vi "FeedbackDecode_KalmanElects2Str.vi"(1 "KalmanElects":T1(array[cluster])) -> (0 "KElectStr":string)   [LabVIEW 2020]
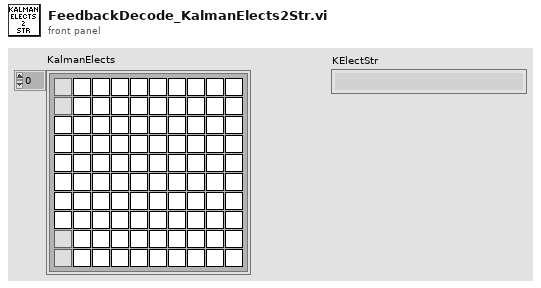
[diagram p1: front panel]
types:
  T1 = cluster{"Boolean 1":bool, "Boolean 2":bool, "Boolean 3":bool, "Boolean 4":bool, "Boolean 5":bool, "Boolean 6":bool, "Boolean 7":bool, "Boolean 8":bool, "Boolean 9":bool, "Boolean 10":bool, "Boolean 11":bool, "Boolean 12":bool, "Boolean 13":bool, "Boolean 14":bool, "Boolean 15":bool, "Boolean 16":bool, "Boolean 17":bool, "Boolean 18":bool, "Boolean 19":bool, "Boolean 20":bool, "Boolean 21":bool, "Boolean 22":bool, "Boolean 23":bool, "Boolean 24":bool, "Boolean 25":bool, "Boolean 26":bool, "Boolean 27":bool, "Boolean 28":bool, "Boolean 29":bool, "Boolean 30":bool, "Boolean 31":bool, "Boolean 32":bool, "Boolean 33":bool, "Boolean 34":bool, "Boolean 35":bool, "Boolean 36":bool, "Boolean 37":bool, "Boolean 38":bool, "Boolean 39":bool, "Boolean 40":bool, "Boolean 41":bool, "Boolean 42":bool, "Boolean 43":bool, "Boolean 44":bool, "Boolean 45":bool, "Boolean 46":bool, "Boolean 47":bool, "Boolean 48":bool, "Boolean 49":bool, "Boolean 50":bool, "Boolean 51":bool, "Boolean 52":bool, "Boolean 53":bool, "Boolean 54":bool, "Boolean 55":bool, "Boolean 56":bool, "Boolean 57":bool, "Boolean 58":bool, "Boolean 59":bool, "Boolean 60":bool, "Boolean 61":bool, "Boolean 62":bool, "Boolean 63":bool, "Boolean 64":bool, "Boolean 65":bool, "Boolean 66":bool, "Boolean 67":bool, "Boolean 68":bool, "Boolean 69":bool, "Boolean 70":bool, "Boolean 71":bool, "Boolean 72":bool, "Boolean 73":bool, "Boolean 74":bool, "Boolean 75":bool, "Boolean 76":bool, "Boolean 77":bool, "Boolean 78":bool, "Boolean 79":bool, "Boolean 80":bool, "Boolean 81":bool, "Boolean 82":bool, "Boolean 83":bool, "Boolean 84":bool, "Boolean 85":bool, "Boolean 86":bool, "Boolean 87":bool, "Boolean 88":bool, "Boolean 89":bool, "Boolean 90":bool, "Boolean 91":bool, "Boolean 92":bool, "Boolean 93":bool, "Boolean 94":bool, "Boolean 95":bool, "Boolean 96":bool, "Boolean 97":bool, "Boolean 98":bool, "Boolean 99":bool, "Boolean 100":bool}[]
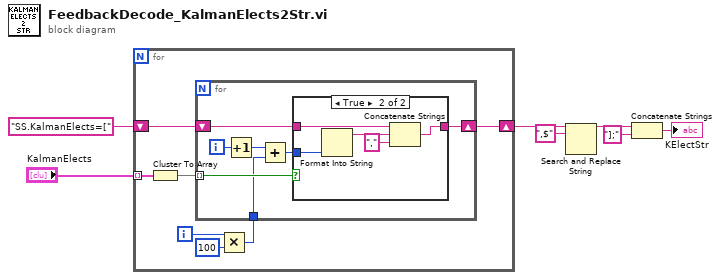
[diagram p0: block diagram]
diagram:
  n1 = for {
    tunnel: "KalmanElects" -> [w13] mode=indexing
    shift-right: [w11] -> w4
    shift-left: "SS.KalmanElects=[" ("string") -> [w12]
    i -> [w10]
    n2 = Cluster To Array(cluster=w13) -> (array=w14:bool[])
    n3 = Multiply(x=w10, y=100) -> (x*y=w8:i32)
    n4 = for {
      shift-right: [w20] -> w11
      shift-left: w12 -> [w21]
      tunnel: w14 -> [w18] mode=indexing
      tunnel: w8 -> [w16]
      i -> [w19]
      n5 = Increment(x=w19) -> (x+1=w17:i32)
      n6 = Add(x=w17, y=w16) -> (x+y=w15:i32)
      n7 = case shown="True" w18 {
        tunnel: w21 -> [w22 w27]
        tunnel: [w22 w26] -> w20
        tunnel: w15 -> [_ w23]
        frame False {
        }
        frame True {
          n8 = Format Into String(w23) -> (resulting string=w25:string)  [unwired: 3 in, 1 out]
          n9 = Concatenate Strings(w27, w25, "," ("string")) -> (w26:string)
        }
      }
    }
  }
  n10 = Search and Replace String(input string=w4, search string=",$") -> (result string=w6:string)  [unwired: 6 in, 3 out]
  n11 = Concatenate Strings(w6, "];" ("string")) -> (→"KElectStr":string)
